vi "TS DAC Acq Start.vi"(8 "error in (no error)":errorcluster, 11 "LNG Boiling Test Stand in":refnum<class "LNG Boiling Test Stand.lvclass">) -> (0 "error out":errorcluster, 3 "LNG Boiling Test Stand out":refnum<class "LNG Boiling Test Stand.lvclass">)   [LabVIEW 2019, in "Test Stands.lvlib" / "LNG Boiling Test Stand.lvclass"]
uses:
  LNG Boiling Test Stand.lvclass
  LNG Boiling Test Stand.lvclass/LNG Boiling Test Stand.ctl
  <vilib>/DAQmx/write.llb/DAQmx Write (Analog DBL 1Chan 1Samp).vi
  <vilib>/DAQmx/miscellaneous.llb/DAQmx Fill In Error Info.vi
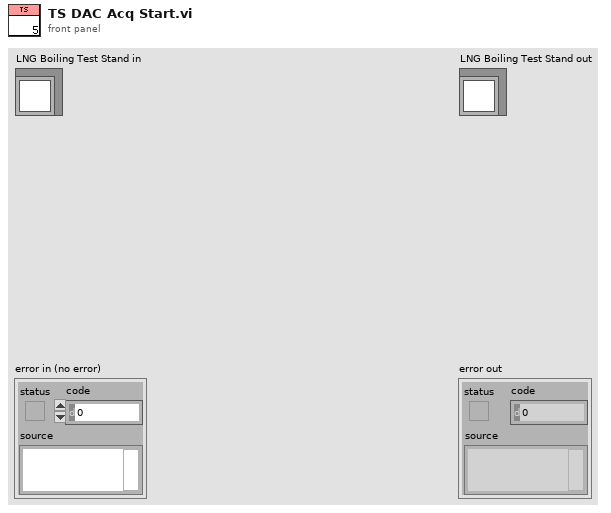
[diagram p1: front panel]
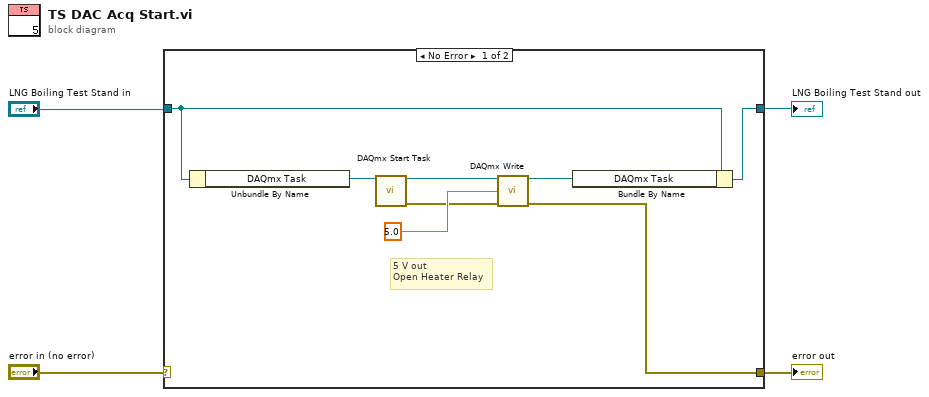
[diagram p0: block diagram]
diagram:
  n1 = case shown="No Error" "error in (no error)" {
    selector: "error in (no error)" -> [_ w14]
    tunnel: [w5 w14] -> w1
    tunnel: [w6 w13] -> w3
    tunnel: "LNG Boiling Test Stand in" -> [w8 w13]
    frame No Error {
      # "5 V out\nOpen Heater Relay"
      n2 = Unbundle By Name(w8) -> ("DAQmx Task"=w12:refnum<k21>)
      n3 = call <vilib>:"DAQmx Start Task.vi"("task/channels in"=w12) -> ("task out"=w11:refnum<k21>, "error out"=w9:errorcluster)  [unwired: 13 in]
      n4 = call-poly <vilib>:"DAQmx Write.vi"("task/channels in"=w11, "data"=5.0, "error in"=w9) -> ("task out"=w7:refnum<k21>, "error out"=w5:errorcluster)  [unwired: 10 in, 1 out]
      n5 = Bundle By Name(cluster=w8, "DAQmx Task"=w7) -> (w6:refnum<class "LNG Boiling Test Stand.lvclass">)
    }
    frame Error {
    }
  }
  "error out" <- w1
  "LNG Boiling Test Stand out" <- w3
